vi "ASE_MPC_Experiment_template.vi"() -> ()   [LabVIEW 2018]
uses:
  <vilib>/Simulation/Implementation/XNodeFramework/SimXNode/SimX.xnode
  <vilib>/Simulation/Implementation/Shared/SIMSCR Execution Mode.ctl
  <vilib>/Simulation/Scripting/Companion Diagram/SimConfigNode/_simSolvers.ctl
  <vilib>/Simulation/Scripting/Companion Diagram/SimConfigNode/SimParams.ctl
  <vilib>/Simulation/Scripting/Companion Diagram/SimConfigNode/SimDog.xnode
  <vilib>/Simulation/ContinuousLinear/Implementation/NILVSim Transfer Function.llb/SIM Transfer Function (SISO).vi
  <vilib>/Simulation/Utility/Implementation/SIM Halt.vi
  <vilib>/Simulation/Nonlinear/Implementation/NILVSim RateLimiter.llb/SIM RateLimiter (scalar).vi
  <vilib>/Simulation/Nonlinear/Implementation/NILVSim Saturation.llb/SIM Saturation (scalar).vi
  <vilib>/Simulation/DataSources/Implementation/NILVSim Signal Generator.llb/SIM Signal Generator (scalar).vi
  <vilib>/Simulation/SignalArithmetic/Implementation/NILVSim Gain.llb/SIM Gain (scalar).vi
  <vilib>/Simulation/Nonlinear/Implementation/NILVSim Saturation.llb/SIM Saturation (vector).vi
  <vilib>/Simulation/ContinuousLinear/Implementation/NILVSim Integrator new.llb/SIM Integrator (scalar).vi
  <vilib>/rvi/interface/nirviReadWriteControl/nirviReadWriteControl.xnode
  <vilib>/rvi/interface/Simulation/niFpgaSimulationCallBeginRW.vi
  <vilib>/rvi/errors/niLvFpgaAdjustHostInterfaceError.vi
  <vilib>/Quanser/Rapid Control Prototyping Toolkit/discrete/CL Bias Removal.vi
  <vilib>/Quanser/Rapid Control Prototyping Toolkit/discrete/_TypeSpecific/CL Bias Removal (Scalar).vi
  <vilib>/Simulation/SignalArithmetic/Implementation/NILVSim Gain.llb/SIM Gain (vector).vi
  NiFpgaLv.dll
  <vilib>/Utility/error.llb/Error Cluster From Error Code.vi
  <vilib>/rvi/interface/nirviCloseFPGA/nirviCloseFPGA.xnode
  <vilib>/FPGAPlugInAG/Dynamic/niLvFpga_Close_Dynamic.vi
  <vilib>/imath/engines/lvmath2/RunTimeEngine/ErrorHandling/NIMS_Create Error From Enums.vi
  <vilib>/imath/engines/lvmath2/RunTimeEngine/ErrorHandling/NIMS_Finalize Error.vi
  <vilib>/imath/engines/lvmath2/RunTimeEngine/BuiltInFunctions/fmin_qp/NIMS_fmin_qp.vi
  <vilib>/imath/engines/lvmath2/RunTimeSupport/NIMS_Complex To Real.vi
  <vilib>/imathl/engines/lvmath/Functions/Error Handling/Create Error.vi
  <vilib>/imath/engines/lvmath2/RunTimeEngine/NodeEndStatement/NIMS_NodeEndStatement_Output.vi
  <vilib>/imath/engines/lvmath2/RunTimeEngine/IndexRead/NIMS V(S).vi
  <vilib>/imath/engines/lvmath2/RunTimeEngine/ArithmeticOperatorToken/NIMS_ArithmeticOperator_multmx.vi
  <vilib>/rvi/interface/nirviOpenFPGA/nirviOpenFPGA.xnode
  <vilib>/addons/Control Design/_Model Construction/NI_LinSys_Model Information.lvlib
  <vilib>/imath/engines/lvmath/Plug In/Control Design/BuiltInFunctions/ss/NIMS_CD_ss(A,B,C,D).vi
  <vilib>/imath/engines/lvmath/Plug In/Control Design/BuiltInFunctions/c_to_d/NIMS_CD_c_to_d(SS,TS,STR,DBL).vi
  <vilib>/imath/engines/lvmath2/RunTimeEngine/ArithmeticOperatorToken/NIMS_ArithmeticOperator_plus.vi
  <vilib>/imath/engines/lvmath2/RunTimeSupport/NIMS_Error if Not Equal.vi
  <vilib>/imath/engines/lvmath2/RunTimeEngine/IndexReplace/NIMS M(S,S)=S.vi
  <vilib>/imath/engines/lvmath2/RunTimeEngine/BuiltInFunctions/eye/NIMS_M=eye(I32, I32).vi
  <vilib>/imath/engines/lvmath2/RunTimeEngine/RangeToken/NIMS_Range_R2 - Float.vi
  <vilib>/imath/engines/lvmath2/RunTimeEngine/CommandStatement/MC_CommandStatement_break.vi
  <vilib>/imath/engines/lvmath2/RunTimeEngine/ArithmeticOperatorToken/NIMS_ArithmeticOperator_powermx(M,M).vi
  <vilib>/imath/engines/lvmath2/RunTimeEngine/MatrixToken/NIMS_MatrixToken_M_M.vi
  <vilib>/imath/engines/lvmath2/RunTimeEngine/BuiltInFunctions/diag/NIMS_diag.vi
  <vilib>/imath/engines/lvmath2/RunTimeEngine/IndexRead/NIMS V(R2).vi
  <vilib>/imath/engines/lvmath2/RunTimeEngine/IndexReplace/NIMS M(V,$)=M.vi
  <vilib>/imath/engines/lvmath2/RunTimeEngine/RangeToken/NIMS_Range.vi
  <vilib>/imath/engines/lvmath2/RunTimeEngine/IndexReplace/NIMS M(R2,R2)=M.vi
  <vilib>/imath/engines/lvmath2/RunTimeEngine/RowToken/NIMS_RowToken_M_M.vi
  <vilib>/addons/Control Design/_Model Construction/Model Information.llb/Model Information SubVIs/cd_Get Matrices From SS Model.vi
  <vilib>/imath/engines/lvmath2/RunTimeEngine/ArithmeticOperatorToken/NIMS_ArithmeticOperator_multmx(M,CV).vi
  <vilib>/imath/engines/lvmath2/RunTimeSupport/NIMS_Get Any Vector_w Error - Matrix.vi
  FPGA Bitfiles/ActiveSuspension_FPGATarget_FPGAQ1MODULE_-QPaFzs6Ihw.lvbitx
  FPGA_Q1_MODULE.vi
  <vilib>/FPGAPlugInAG/cRIO-9068/niLvFpga_Open_cRIO-9068.vi
  <vilib>/rvi/interface/common/dynamic/niFpgaDynamicAddResources.vi
panel:
  in  "weight O4":dbl
  in  "weight O3":dbl
  in  "weight I1":dbl
  in  "weight O2":dbl
  in  "weight O1":dbl
  in  "Control Horizon (Nc)":u64 step=1
  in  "Prediction Horizon (Np)":u64 step=1
  in  "Enable motor":bool
  in  "Setpoint Command 2":T1={"Amplitude (m)"=0.01, "Frequency (Hz)"=0.3} caption="Road (Bottom Plate)\nAmplitude Command (m)" {"Frequency (Hz)" min=0.0 max=0.5 step=0.009999999776482582 format="%_3f"; "Amplitude (m)" min=-10.0 max=10.0 step=0.5 format="%_3f"}
  out "Active Suspension Motor Voltage (V)":dbl(graph)
  in  "Enable active suspension":bool
  out "Zr(m), Zs(m), Zus(m) 2":T2(graph)={"output"=0.0096065956, "Result"=0.0090666584, "output"=0.0091514816}
  out "Accelerometer Signal":dbl(graph)
  in  "Halt?":bool
  # "Active Suspension MPC"
  # "MPC parameters"
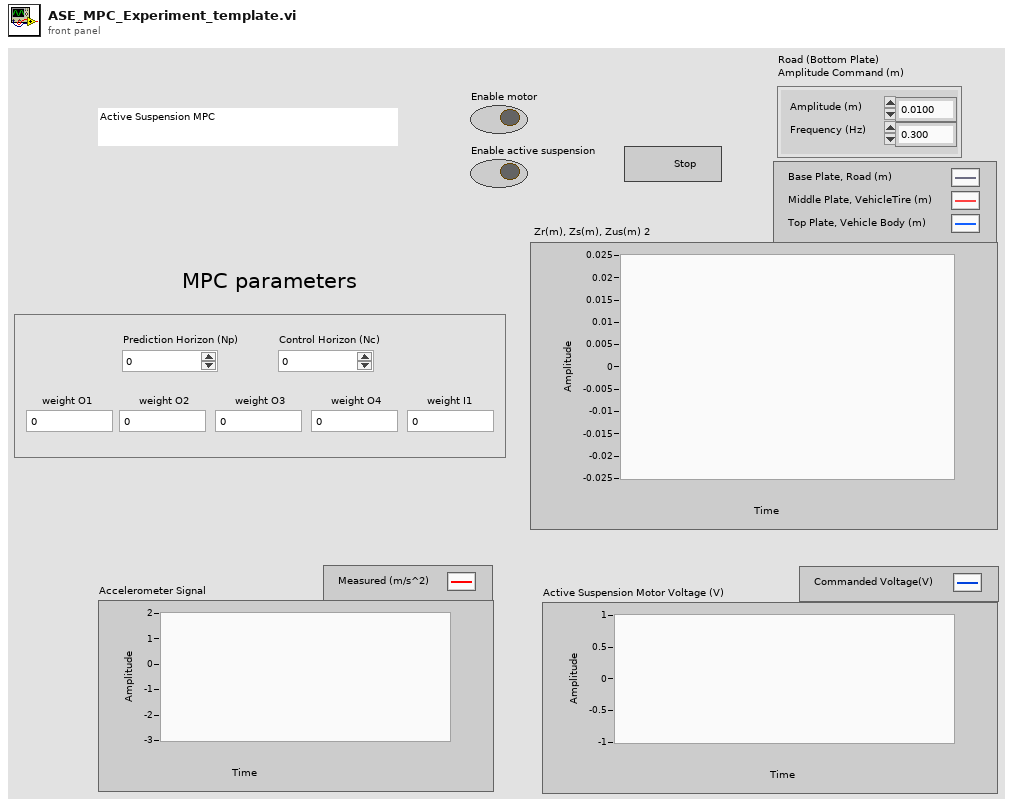
[diagram p1: front panel]
types:
  T1 = cluster{"Amplitude (m)":dbl, "Frequency (Hz)":dbl}
  T2 = cluster{"output":dbl, "Result":dbl, "output":dbl}
  T3 = typedef "SimParams.ctl" = cluster{"Initial Time (s)":dbl, "Final Time (s)":dbl, "Step Size (s)":dbl, "ODE Solver":T4, "Minimum Step Size (s)":dbl, "Maximum Step Size (s)":dbl, "Relative Tolerance":dbl, "Absolute Tolerance":dbl, "Software Timing":bool, "Initial Step Size (s)":dbl, "Automatic Fixed Step Size?":bool, "Automatic Discrete Step Size?":bool, "Discrete Step Size (s)":dbl, "Calculate using Time Step":bool, "Solver Wired?":bool, "Prev.Frm.Expected End":u64, "Prev.Frm.Actual End":u64, "Prev.Frm.Finished Late?":bool, "Prev.Iter.Expected End":u64, "Prev.Iter.Actual End":u64, "Prev.Iter.Finished Late?":bool, "Expected Iteration Start":u64, "Actual Iteration Start":u64, "Expected Frame Start":u64, "Actual Frame Start":u64, "Source Name":string, "Name":string, "Period":i64, "Deadline":i64, "Offset":i64, "Start":i64, "Priority":i32, "Timeout":i32, "Processor":i32, "Mode":enum32{"No Change", "Process missed periods, maintain original phase", "Discard missed periods, maintain original phase", "Process missed periods, ignore original phase", "Discard missed periods, ignore original phase"}, "Wakeup reason":enum32{"Normal", "Aborted", "Asynchronous wakeup", "Timing source error", "Timed loop error", "Timeout"}, "Error":errorcluster, "Source Type":string, "Secondary Source Type":string, "Global End Time":u64, "Global Start Time":u64, "Full Solver Reset":bool, "Execution Mode":T5, "Nan/Inf Check":bool, "Custom Solver Library":string, "Solver Is Variable":bool, "custom solver name":string, "Signal Collection Decimation":u32}
  T4 = typedef "_simSolvers.ctl" = enum16{"Runge-Kutta 1 (Euler)", "Runge-Kutta 2", "Runge-Kutta 3", "Runge-Kutta 4", "Runge-Kutta 23 (variable)", "Runge-Kutta 45 (variable)", "BDF (variable)", "Adams-Moulton (variable)", "Rosenbrock (variable)", "Discrete States Only", "SDIRK 4 (variable)", "Radau 5 (variable)", "Radau 9 (variable)", "Radau 13 (variable)", "Radau [Variable Order] (variable)", "Gear's Method (variable)", "Linearizer", "State Query", "Trim Eval", "Custom Solver"}
  T5 = typedef "SIMSCR Execution Mode.ctl" = enum16{"Simulate to Completion", "Single Time-Step Simulation (Fixed Step Only)"}
  T6 = typedef "NI_LinSys_Model Typedefs.lvlib/CD State Space Model (MIMO).ctl" = cluster{"properties":T7, "A":dbl[][], "B":dbl[][], "C":dbl[][], "D":dbl[][], "StateNames":string[], "Transport Delay":dbl[][]}
  T7 = typedef "NI_LinSys_Model Typedefs.lvlib/CD General Elements.ctl" = cluster{"Model name":string, "Input names":string[], "Output names":string[], "Input Delays":dbl[], "Output Delays":dbl[], "Sampling Time":dbl, "Notes":string}
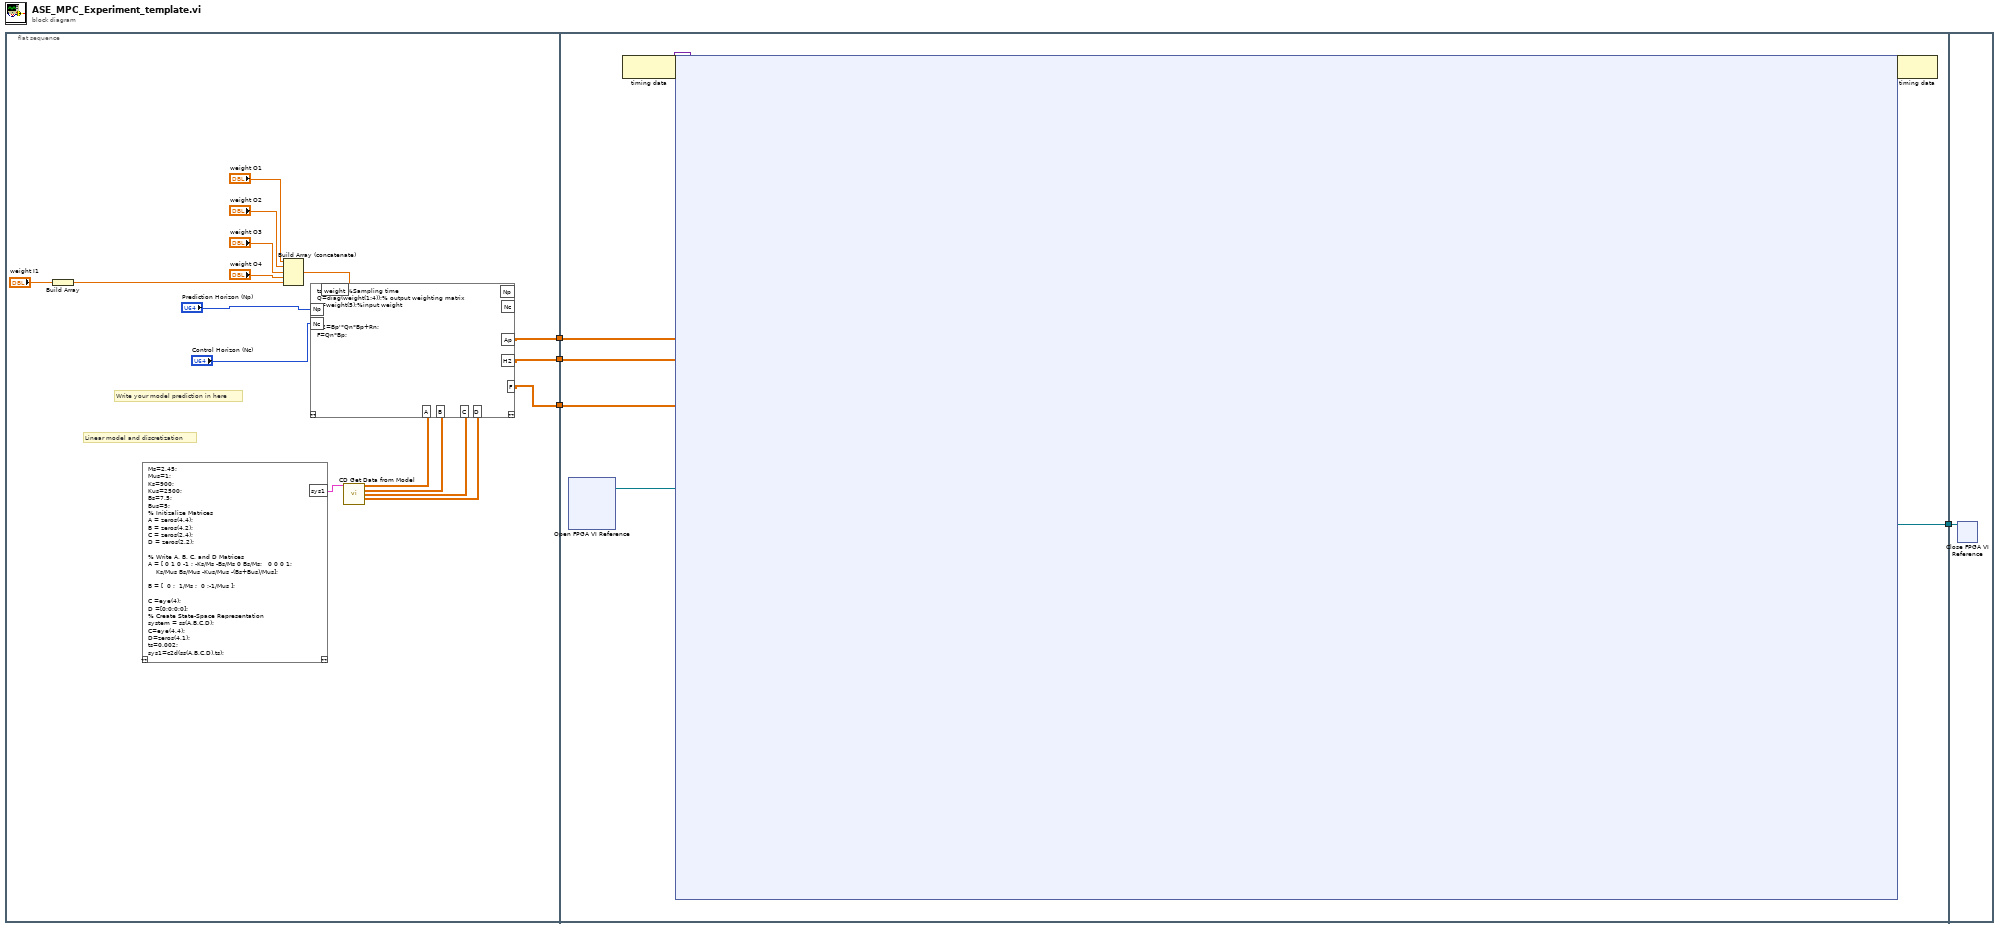
[diagram p0: block diagram]
diagram:
  n1 = flat-sequence {
    tunnel: [w14] -> w3
    tunnel: [w13] -> w2
    tunnel: [w12] -> w1
    tunnel: [w789] -> w4
    tunnel: w3 -> [w788]
    tunnel: w2 -> [w787]
    tunnel: w1 -> [w786]
    tunnel: w4 -> [w1099]
    frame #0 {
      # "Write your model prediction in here"
      # "Linear model and discretization"
      n2 = Build Array ("Build Array 4")("weight I1") -> (w18:dbl[])
      n3 = mathscript code="Ms=2.45;\nMus=1;\nKs=900;\nKus=2500;\nBs=7.5;\nBus=5;\n% Initizalize Matrices\nA = zeros(4,4);\nB = zeros(4,2);\nC = zeros(2,4);\nD = zeros(2,2);\n\n% Write A, B, C, and D Matrices\nA = [ 0 1 0 -1 ; -Ks/Ms -Bs/Ms 0 Bs/Ms;   0 0 0 1;\n    Ks/Mus Bs/Mus -Kus/Mus -(Bs+Bus)/Mus];\n\nB = [  0 ;  1/Ms ;  0 ;-1/Mus ];\n\nC =eye(4);\nD =[0;0;0;0];\n% Create State-Space Representation\nsystem = ss(A,B,C,D);\nC=eye(4,4);\nD=zeros(4,1);\nts=0.002;\nsys1=c2d(ss(A,B,C,D),ts);"() -> ("sys1"=w11:T6)  [unwired: 1 in, 1 out]
      n4 = Build Array (concatenate) ("Build Array 3")("weight O1", "weight O2", "weight O3", "weight O4", w18) -> (w17:dbl[])
      n5 = call-poly <vilib>:"CD Get Data from Model.vi"("State-Space Model"=w11) -> ("Matrix A"=w10:dbl[][], "Matrix B"=w8:dbl[][], "Matrix C"=w9:dbl[][], "Matrix D"=w7:dbl[][])  [unwired: 10 in, 1 out]
      n6 = mathscript code="ts=0.002;%Sampling time\nQ=diag(weight(1:4));% output weighting matrix\nR=weight(5);%input weight\n\n\nH2=Bp'*Qn*Bp+Rn;\nF=Qn*Bp;" ("MathScript Node 2")("Np"="Prediction Horizon (Np)", "Nc"="Control Horizon (Nc)", "weight"=w17, "A"=w10, "B"=w8, "C"=w9, "D"=w7) -> ("Np"=w16:dbl, "Nc"=w15:dbl, "Ap"=w14:cdb[][], "F"=w12:cdb[][], "H2"=w13:cdb[][])  [unwired: 1 in, 1 out]
    }
    frame #1 {
      n7 = xnode "Open FPGA VI Reference"() -> ("FPGA VI Reference Out"=w790:refnum<k20>)  [unwired: 2 in, 1 out]
      n8 = node-c288() -> (w792:variant)  [unwired: 1 in]
      n9 = node-c254 ("Control & Simulation Loop")(w792, w790, w788, w787, w786) -> (w791:variant, w789:refnum<k20>)
      n10 = node-c288(w791) -> ()  [unwired: 1 out]
    }
    frame #2 {
      n11 = xnode "Close FPGA VI Reference"("FPGA VI Reference In"=w1099) -> ()  [unwired: 1 in, 1 out]
    }
  }
